vi "Limit Page DOF Names 2 Text.vi"(10 "DofType":T1) -> (2 "Transactions":string[](array[string]))   [LabVIEW 2013]
uses:
  Data Access Objects/Limits/DofTypes.ctl
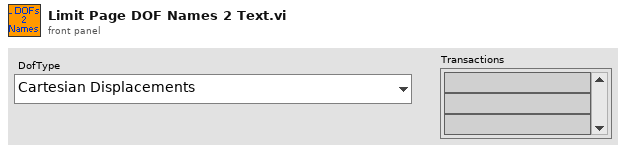
[diagram p1: front panel]
types:
  T1 = typedef "DofTypes.ctl" = enum16{"Cartesian Displacements", "Cartesian Forces & Moments", "Actuator Displacements", "Actuator Forces", "Cartesian Increments", "Actuator Increments"}
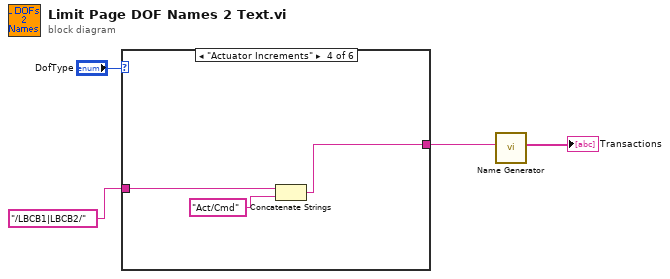
[diagram p0: block diagram]
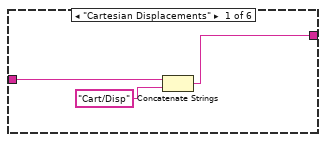
[diagram p2: hidden frame]
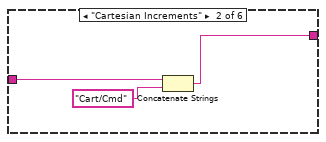
[diagram p3: hidden frame]
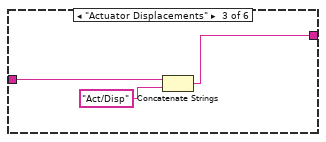
[diagram p4: hidden frame]
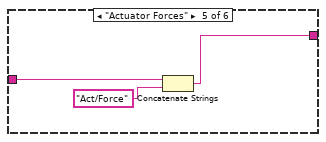
[diagram p5: hidden frame]
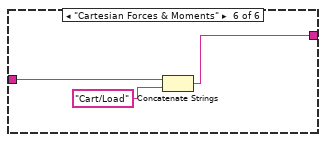
[diagram p6: hidden frame]
diagram:
  n1 = case shown="\"Actuator Increments\"" "DofType" {
    tunnel: "/LBCB1|LBCB2/" -> [w7 w10 w13 w16 w19 w22]
    tunnel: [w5 w8 w11 w14 w17 w20] -> w1
    frame "Cartesian Displacements" {
      n2 = Concatenate Strings(w7, "Cart/Disp" ("string")) -> (w5:string)
    }
    frame "Cartesian Increments" {
      n3 = Concatenate Strings(w10, "Cart/Cmd" ("string")) -> (w8:string)
    }
    frame "Actuator Displacements" {
      n4 = Concatenate Strings(w13, "Act/Disp" ("string")) -> (w11:string)
    }
    frame "Actuator Increments" {
      n5 = Concatenate Strings(w16, "Act/Cmd" ("string")) -> (w14:string)
    }
    frame "Actuator Forces" {
      n6 = Concatenate Strings(w19, "Act/Force" ("string")) -> (w17:string)
    }
    frame "Cartesian Forces & Moments" {
      n7 = Concatenate Strings(w22, "Cart/Load" ("string")) -> (w20:string)
    }
  }
  n8 = call "Name Generator.vi"("Group Specifier"=w1) -> ("Group Names"=→"Transactions":string[])  [unwired: 10 in]
